vi "PH_Beckhoff_PP_Control.ProcCases.vi"(0 "i ref in":refnum<vi>, 1 "selector":string, 2 "Data":T1, 3 "call cluster":T2={"Object"="", "Selector"="", "CallType"=enum."synchronous", "Async Object"="", "Async Selector"="", "Data Descriptor"="", "Data"=[], "Error #"=0, "Expire"=0}, 5 "error in (no error)":errorcluster) -> (14 "i ref out":refnum<vi>, 17 "answer cluster":T2={"Object"="", "Selector"="", "CallType"=enum."synchronous", "Async Object"="", "Async Selector"="", "Data Descriptor"="", "Data"=[], "Error #"=0, "Expire"=0}, 19 "error out":errorcluster)   [LabVIEW 2014, in "PH_Beckhoff_PP_Control.lvlib"]
doc: "This method is called by a process from within the default case in the event loop. The methods of a class that are linked to events will be called from THIS method. Add your code here."
uses:
  PH_Beckhoff_PP_Control.lvlib
  CSCore/CSSystem/CoreDefs/CoreDefs.call_type.ctl
  CSCore/BaseProcess/BaseProcess.descriptor string definition.ctl
  CSCore/CSSystem/CoreDefs/CoreDefs.rawDataType.ctl
  CSCore/CSSystem/CoreLib/CoreLib.string 2 byte array.vi
  PH_Beckhoff/PH_Beckhoff.lvlib
  CSCore/CSSystem/CoreLib/CoreLib.lvlib
  CSCore/BaseProcess/BaseProcess.lvlib
  CSCore/CAEObj/CAEObj.lvlib
  PH_PSDBWriter/PH_PSDBWriter.lvlib
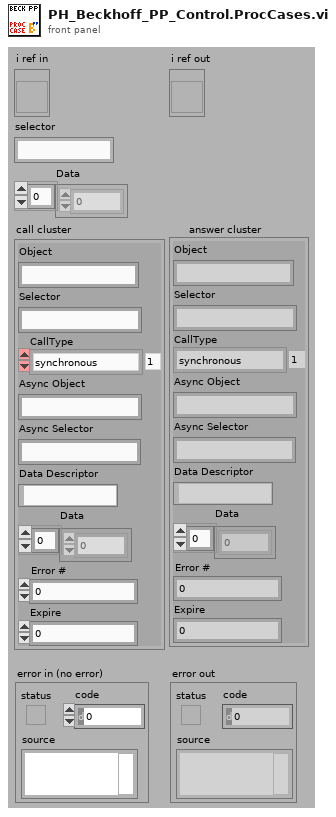
[diagram p1: front panel]
types:
  T1 = typedef "CoreDefs.rawDataType.ctl" = i8[]
  T2 = typedef "CoreDefs.call_type.ctl" = cluster{"Object":string, "Selector":string, "CallType":enum16{"simple", "synchronous", "asynchronous"}, "Async Object":string, "Async Selector":string, "Data Descriptor":T3, "Data":T1, "Error #":i32, "Expire":u32}
  T3 = typedef "BaseProcess.lvlib/BaseProcess.descriptor string definition.ctl" = string
  T4 = typedef "PH_Beckhoff_PP_Control.lvlib/PH_Beckhoff_PP_Control.i attribute.ctl" = cluster{"PP Conductivity Control":cluster{"PSDB":cluster{"Status Service ID":i32, "Instance ID":i32, "Data Status":T5, "Ref Status":refnum<vi>, "Error Code":i32}, "Status":cluster{"GUI Ref":refnum<vi>, "Status Service ID":i32, "Status":T6}, "DIs":cluster{"Device on":cluster{"GUI Ref":refnum<vi>, "# in Data":i32}, "Conductivity ok":cluster{"GUI Ref":refnum<vi>, "# in Data":i32}, "Temperature ok":cluster{"GUI Ref":refnum<vi>, "# in Data":i32}, "Alarm":cluster{"GUI Ref":refnum<vi>, "# in Data":i32}}, "PSDB Thread":cluster{"Ref":refnum<vi>, "Q-Ref":refnum<queue>}}, "PP Mercury Control":cluster{"PSDB":cluster{"Status Service ID":i32, "Instance ID":i32, "Data Status":T5, "Ref Status":refnum<vi>, "Error Code":i32}, "Status":cluster{"GUI Ref":refnum<vi>, "Status Service ID":i32, "Status":T6}, "on since:":cluster{"GUI Ref":refnum<vi>, "Service ID":i32, "Time":string}, "DIs":cluster{"Device on":cluster{"GUI Ref":refnum<vi>, "# in Data":i32}, "Alarm":cluster{"GUI Ref":refnum<vi>, "# in Data":i32}}, "AIs":cluster{"Concentration":cluster{"GUI Ref":refnum<vi>, "# in Data":i32}}, "PSDB Thread":cluster{"Ref":refnum<vi>, "Q-Ref":refnum<queue>}}, "PSDB":cluster{"Shot #":i32, "Subsystem":T7}, "PSDB Credentials":T8}
  T5 = typedef "PH_PSDBWriter.lvlib/PH_PSDBWriter.Data Status.ctl" = i16
  T6 = typedef "PH_StatusHandler.lvlib/PH_StatusHandler.Status.ctl" = i16
  T7 = typedef "PH_PSDBWriter.lvlib/PH_PSDBWriter.PHELIX-Subsystems.ctl" = i32
  T8 = typedef "PH_Common.lvlib/PH_Connection.PSDB Credentials.ctl" = cluster{"PW":string, "ID":string, "DS":string}
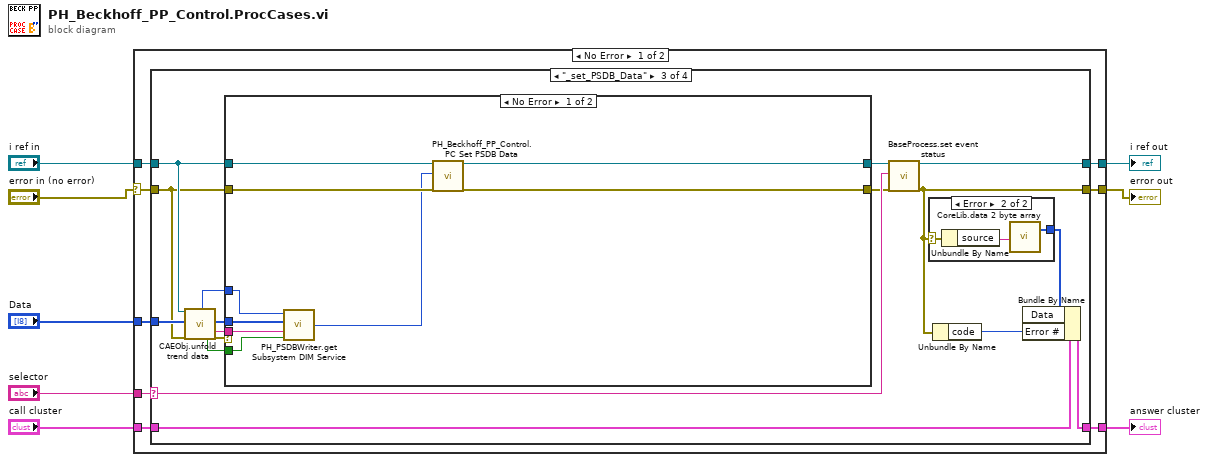
[diagram p0: block diagram]
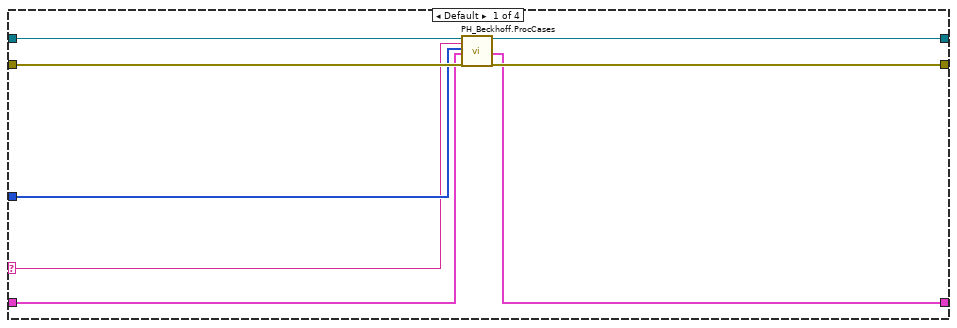
[diagram p2: hidden frame]
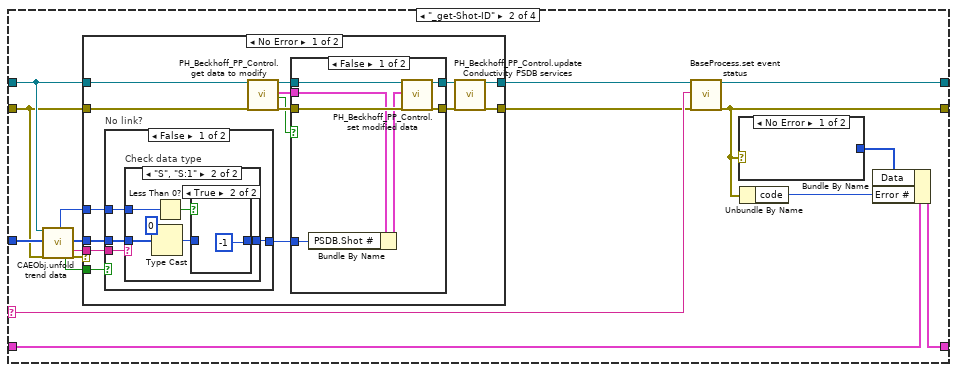
[diagram p3: hidden frame]
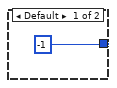
[diagram p5: hidden frame]
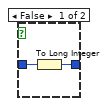
[diagram p6: hidden frame]
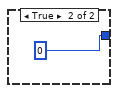
[diagram p7: hidden frame]
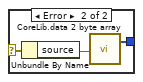
[diagram p9: hidden frame]
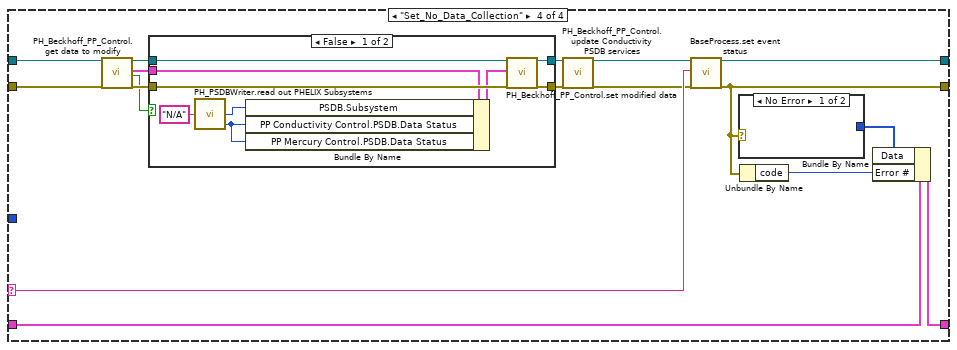
[diagram p12: hidden frame]
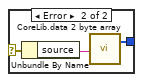
[diagram p14: hidden frame]
diagram:
  n1 = case shown="No Error" "error in (no error)" {
    selector: "error in (no error)" -> [w9 w148]
    tunnel: "selector" -> [w16 _]
    tunnel: [w15 w149] -> w7
    tunnel: "Data" -> [w14 _]
    tunnel: "call cluster" -> [w13 w149]
    tunnel: "i ref in" -> [w12 w150]
    tunnel: [w11 w150] -> w3
    tunnel: [w10 w148] -> w2
    frame No Error {
      n2 = case shown="\"_set_PSDB_Data\"" w16 {
        selector: w16 -> [w18 w37 w98 w129]
        tunnel: w14 -> [w19 w31 w92 _]
        tunnel: w12 -> [w17 w30 w91 w126]
        tunnel: [w24 w39 w100 w131] -> w11
        tunnel: w13 -> [w20 w36 w97 w128]
        tunnel: [w21 w35 w96 w127] -> w15
        tunnel: w9 -> [w23 w27 w88 w123]
        tunnel: [w22 w38 w99 w130] -> w10
        frame Default {
          n3 = call "PH_Beckhoff.ProcCases.vi"("i ref in"=w17, "selector"=w18, "Data"=w19, "call cluster"=w20, "error in (no error)"=w23) -> ("i ref out"=w24:refnum<vi>, "answer cluster"=w21:T2, "error out"=w22:errorcluster)  [unwired: 12 in]
        }
        frame "_get-Shot-ID" {
          n4 = call "CAEObj.unfold trend data.vi"("i ref in"=w30, "raw trend data"=w31, "error in (no error)"=w27) -> ("quality"=w32:i32, "no link"=w34:bool, "data"=w26:i8[], "typeDescriptor"=w25:string, "error out"=w33:errorcluster)  [unwired: 8 in, 4 out]
          n5 = case shown="No Error" w33 {
            tunnel: w27 -> [w52 w82]
            tunnel: [w45 w81] -> w29
            tunnel: [w43 w82] -> w28
            tunnel: w30 -> [w51 w81]
            tunnel: w34 -> [w56 _]
            tunnel: w25 -> [w55 _]
            tunnel: w26 -> [w54 _]
            tunnel: w32 -> [w53 _]
            frame No Error {
              n6 = case "No link?" shown="False" w56 {
                tunnel: [w69 0] -> w46
                tunnel: w53 -> [w68 _]
                tunnel: w54 -> [w67 _]
                tunnel: w55 -> [w66 _]
                frame False {
                  n7 = case "Check data type" shown="\"S\", \"S:1\"" w66 {
                    tunnel: [-1 w76] -> w69
                    tunnel: w68 -> [_ w74]
                    tunnel: w67 -> [_ w72]
                    frame Default {
                    }
                    frame "S", "S:1" {
                      n8 = Type Cast(type=i16 0, x=w72) -> (*(type *) &x=w71:i16)
                      n9 = Less Than 0?(x=w74) -> (x < 0?=w75:bool)
                      n10 = case shown="True" w75 {
                        tunnel: [w77 -1] -> w76
                        tunnel: w71 -> [w78 _]
                        frame False {
                          n11 = To Long Integer(number=w78) -> (32bit integer=w77:i32)
                        }
                        frame True {
                        }
                      }
                    }
                  }
                }
                frame True {
                }
              }
              n12 = call "PH_Beckhoff_PP_Control.get data to modify.vi"("i ref in"=w51, "error in (no error)"=w52) -> ("i ref out"=w49:refnum<vi>, "i attribute"=w47:T4, "timed out"=w48:bool, "error out"=w50:errorcluster)  [unwired: 14 in]
              n13 = case shown="False" w48 {
                tunnel: w50 -> [w63 w64]
                tunnel: [w62 w64] -> w42
                tunnel: w49 -> [w61 w65]
                tunnel: [w60 w65] -> w44
                tunnel: w47 -> [w59 _]
                tunnel: w46 -> [w57 _]
                frame False {
                  n14 = Bundle By Name(cluster=w59, "PSDB.Shot #"=w57) -> (w58:T4)
                  n15 = call "PH_Beckhoff_PP_Control.set modified data.vi"("i ref in"=w61, "i attribute"=w58, "error in (no error)"=w63) -> ("i ref out"=w60:refnum<vi>, "error out"=w62:errorcluster)  [unwired: 15 in]
                }
                frame True {
                }
              }
              n16 = call "PH_Beckhoff_PP_Control.update Conductivity PSDB services.vi"("i ref in"=w44, "error in"=w42) -> ("i ref out"=w45:refnum<vi>, "error out"=w43:errorcluster)  [unwired: 16 in]
            }
            frame Error {
            }
          }
          n17 = call "BaseProcess.set event status.vi"("i ref in"=w29, "EventStatus"=w37, "error in (no error)"=w28) -> ("i ref out"=w39:refnum<vi>, "error out"=w38:errorcluster)  [unwired: 14 in, 1 out]
          n18 = case shown="No Error" w38 {
            selector: w38 -> [_ w85]
            tunnel: [_ w83] -> w40
            frame No Error {
            }
            frame Error {
              n19 = Unbundle By Name(w85) -> ("source"=w84:string)
              n20 = call-poly "CoreLib.data 2 byte array.vi"("string"=w84) -> ("byteArray out"=w83:T1)  [unwired: 18 in]
            }
          }
          n21 = Unbundle By Name(w38) -> ("code"=w41:i32)
          n22 = Bundle By Name(cluster=w36, "Data"=w40, "Error #"=w41) -> (w35:T2)
        }
        frame "_set_PSDB_Data" {
          n23 = call "CAEObj.unfold trend data.vi"("i ref in"=w91, "raw trend data"=w92, "error in (no error)"=w88) -> ("quality"=w93:i32, "no link"=w95:bool, "data"=w87:i8[], "typeDescriptor"=w86:string, "error out"=w94:errorcluster)  [unwired: 8 in, 4 out]
          n24 = case shown="No Error" w94 {
            tunnel: w88 -> [w109 w113]
            tunnel: [w108 w112] -> w90
            tunnel: [w111 w113] -> w89
            tunnel: w91 -> [w110 w112]
            tunnel: w95 -> [w103 _]
            tunnel: w86 -> [w105 _]
            tunnel: w87 -> [w106 _]
            tunnel: w93 -> [w104 _]
            frame No Error {
              n25 = call "PH_PSDBWriter.get Subsystem DIM Service.vi"("no link"=w103, "typeDescriptor"=w105, "data"=w106, "quality"=w104) -> ("PHELIX Subsystems"=w107:T7)
              n26 = call "PH_Beckhoff_PP_Control.PC Set PSDB Data.vi"("VI in"=w110, "PHELIX Subsystem"=w107, "error in (no error)"=w109) -> ("VI out"=w108:refnum<vi>, "error out"=w111:errorcluster)  [unwired: 15 in]
            }
            frame Error {
            }
          }
          n27 = call "BaseProcess.set event status.vi"("i ref in"=w90, "EventStatus"=w98, "error in (no error)"=w89) -> ("i ref out"=w100:refnum<vi>, "error out"=w99:errorcluster)  [unwired: 14 in, 1 out]
          n28 = case shown="Error" w99 {
            selector: w99 -> [_ w116]
            tunnel: [_ w114] -> w101
            frame No Error {
            }
            frame Error {
              n29 = Unbundle By Name(w116) -> ("source"=w115:string)
              n30 = call-poly "CoreLib.data 2 byte array.vi"("string"=w115) -> ("byteArray out"=w114:T1)  [unwired: 18 in]
            }
          }
          n31 = Unbundle By Name(w99) -> ("code"=w102:i32)
          n32 = Bundle By Name(cluster=w97, "Data"=w101, "Error #"=w102) -> (w96:T2)
        }
        frame "Set_No_Data_Collection" {
          n33 = call "PH_Beckhoff_PP_Control.get data to modify.vi"("i ref in"=w126, "error in (no error)"=w123) -> ("i ref out"=w121:refnum<vi>, "i attribute"=w119:T4, "timed out"=w120:bool, "error out"=w122:errorcluster)  [unwired: 14 in]
          n34 = case shown="False" w120 {
            tunnel: w122 -> [w142 w143]
            tunnel: [w141 w143] -> w117
            tunnel: w121 -> [w140 w144]
            tunnel: [w139 w144] -> w118
            tunnel: w119 -> [w138 _]
            frame False {
              n35 = call "PH_PSDBWriter.read out PHELIX Subsystems.vi"("Config DB Subsystem"="N/A") -> ("Metadata.Data Status"=w135:T5, "Metadata.Subsystem"=w136:T7)  [unwired: 2 in, 1 out]
              n36 = Bundle By Name(cluster=w138, "PSDB.Subsystem"=w136, "PP Conductivity Control.PSDB.Data Status"=w135, "PP Mercury Control.PSDB.Data Status"=w135) -> (w137:T4)
              n37 = call "PH_Beckhoff_PP_Control.set modified data.vi"("i ref in"=w140, "i attribute"=w137, "error in (no error)"=w142) -> ("i ref out"=w139:refnum<vi>, "error out"=w141:errorcluster)  [unwired: 15 in]
            }
            frame True {
            }
          }
          n38 = call "PH_Beckhoff_PP_Control.update Conductivity PSDB services.vi"("i ref in"=w118, "error in"=w117) -> ("i ref out"=w125:refnum<vi>, "error out"=w124:errorcluster)  [unwired: 16 in]
          n39 = call "BaseProcess.set event status.vi"("i ref in"=w125, "EventStatus"=w129, "error in (no error)"=w124) -> ("i ref out"=w131:refnum<vi>, "error out"=w130:errorcluster)  [unwired: 14 in, 1 out]
          n40 = case shown="No Error" w130 {
            selector: w130 -> [_ w147]
            tunnel: [_ w145] -> w132
            frame No Error {
            }
            frame Error {
              n41 = Unbundle By Name(w147) -> ("source"=w146:string)
              n42 = call-poly "CoreLib.data 2 byte array.vi"("string"=w146) -> ("byteArray out"=w145:T1)  [unwired: 18 in]
            }
          }
          n43 = Unbundle By Name(w130) -> ("code"=w133:i32)
          n44 = Bundle By Name(cluster=w128, "Data"=w132, "Error #"=w133) -> (w127:T2)
        }
      }
    }
    frame Error {
    }
  }
  "answer cluster" <- w7
  "i ref out" <- w3
  "error out" <- w2
